vi "Message Into String.vi"(8 "error in (no error)":errorcluster, 11 "iMessage in":refnum<class "iMessage.lvclass">) -> (0 "error out":errorcluster, 1 "String":string, 3 "iMessage out":refnum<class "iMessage.lvclass">)   [LabVIEW 2017, in "Message Interface.lvlib" / "iMessage.lvclass"]
uses:
  iMessage.lvclass
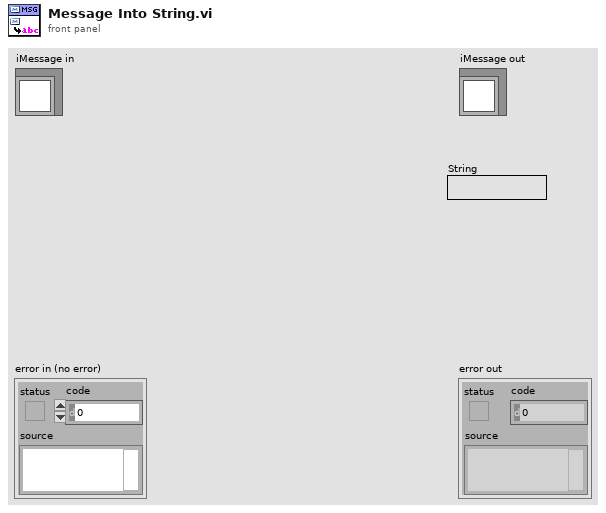
[diagram p1: front panel]
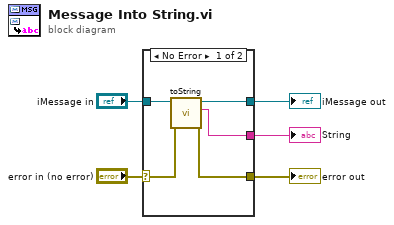
[diagram p0: block diagram]
diagram:
  n1 = case shown="No Error" "error in (no error)" {
    selector: "error in (no error)" -> [w8 w12]
    tunnel: [w7 w12] -> w4
    tunnel: [w9 w11] -> w2
    tunnel: "iMessage in" -> [w10 w11]
    tunnel: [w6 _] -> w1
    frame No Error {
      n2 = call-dynamic "toString.vi"("error in (no error)"=w8, "iMessage in"=w10) -> ("error out"=w7:errorcluster, "String"=w6:string, "iMessage out"=w9:refnum<class "iMessage.lvclass">)  [unwired: 7 in]
    }
    frame Error {
    }
  }
  "error out" <- w4
  "iMessage out" <- w2
  "String" <- w1
